vi "Check Power Source.vi"(8 "error in (no error)":errorcluster, 11 "PicoScope 3000a in":refnum<class "PicoScope 3000a.lvclass">) -> (0 "error out":errorcluster, 3 "PicoScope 3000a out":refnum<class "PicoScope 3000a.lvclass">)   [LabVIEW 2018, in "PicoScope 3000a.lvlib" / "PicoScope 3000a.lvclass"]
uses:
  PicoScope 3000a.lvclass
  PicoScope 3000a.lvclass/PicoScope 3000a.ctl
  <instrlib>/PicoScope/PicoScope.lvlib
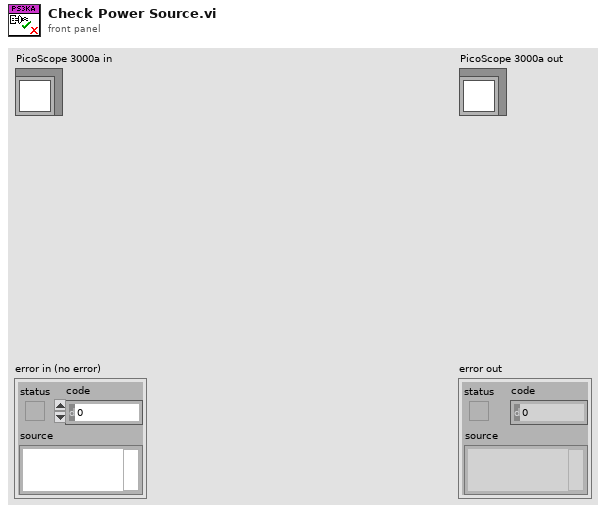
[diagram p1: front panel]
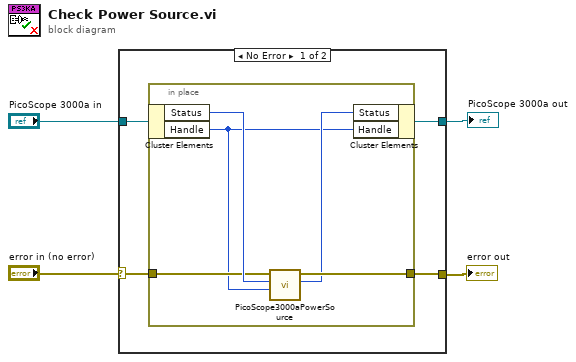
[diagram p0: block diagram]
diagram:
  n1 = case shown="No Error" "error in (no error)" {
    selector: "error in (no error)" -> [w8 w15]
    tunnel: [w7 w15] -> w3
    tunnel: [w5 w14] -> w1
    tunnel: "PicoScope 3000a in" -> [w6 w14]
    frame No Error {
      n2 = in-place {
        in-place-border: w8 -> [w12]
        in-place-border: [w11] -> w7
        n3 = in-place-cluster #1(w6) -> ("Status"=w13:i32, "Handle"=w9:i16)
        n4 = call <instrlib>:"PicoScope3000aPowerSource.vi"("handle in"=w9, "PICO STATUS IN"=w13, "error in (no error)"=w12) -> ("PICO STATUS OUT"=w10:i32, "error out"=w11:errorcluster)  [unwired: 4 in, 3 out]
        n5 = in-place-cluster #1("Status"=w10, "Handle"=w9) -> (w5:refnum<class "PicoScope 3000a.lvclass">)
      }
    }
    frame Error {
    }
  }
  "error out" <- w3
  "PicoScope 3000a out" <- w1
